vi "create_listener.vi"(0 "control_endpoint":string="tcp://0.0.0.0:5556", 5 "Port":string="5555", 7 "recv_timout_default_ms":dbl=2000.0 format="%#_13g", 9 "send_timout_default_ms":dbl=2000.0 format="%#_13g", 11 "error in (no error)":errorcluster) -> (4 "zmq_mlt out":refnum<class "zmq_multipart_lib.lvclass">, 15 "error out":errorcluster)   [LabVIEW 2019, in "zmq_multipart_lib.lvlib" / "zmq_multipart_lib.lvclass"]
uses:
  zmq_multipart_lib.lvclass
  <vilib>/addons/zeromq/socket_type.ctl
  zmq_multipart_lib.lvclass/zmq_multipart_lib.ctl
  <vilib>/addons/zeromq/zmq_context.lvclass
  <vilib>/addons/zeromq/zmq_socket.lvclass
  <vilib>/addons/zeromq/zeromq.lvlib
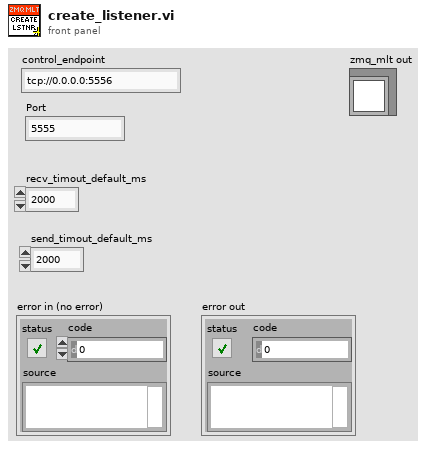
[diagram p1: front panel]
types:
  T1 = typedef "zeromq.lvlib/socket_type.ctl" = enum8{"ZMQ_PAIR", "ZMQ_PUB", "ZMQ_SUB", "ZMQ_REQ", "ZMQ_REP", "ZMQ_DEALER", "ZMQ_ROUTER", "ZMQ_PULL", "ZMQ_PUSH", "ZMQ_XPUB", "ZMQ_XSUB"}
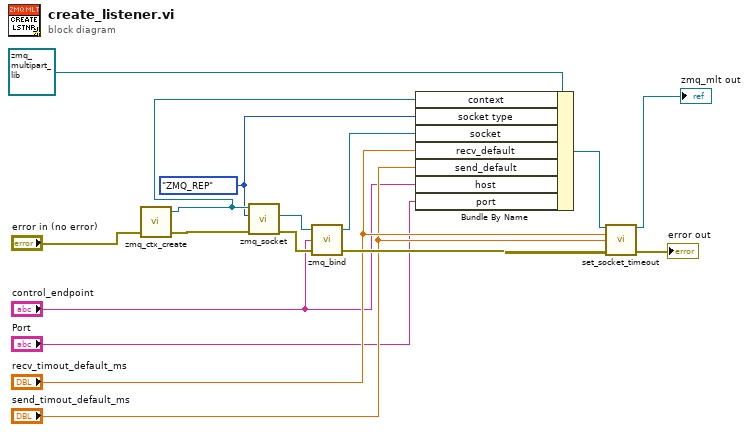
[diagram p0: block diagram]
diagram:
  w7 = socket_type."ZMQ_REP" ("socket type")
  n1 = call <vilib>:"zmq_ctx_create.vi"("error in"="error in (no error)") -> ("error out"=w12:errorcluster, "context out"=w10:refnum<class "zmq_context.lvclass">)  [unwired: 3 in]
  n2 = call <vilib>:"zmq_socket.vi"("error in"=w12, "socket type"=w7, "context in"=w10) -> ("error out"=w14:errorcluster, "socket out"=w6:refnum<class "zmq_socket.lvclass">)  [unwired: 2 in, 1 out]
  n3 = call <vilib>:"zmq_bind.vi"("error in"=w14, "endpoint"="control_endpoint", "socket in"=w6) -> ("error out"=w15:errorcluster, "socket out"=w5:refnum<class "zmq_socket.lvclass">)  [unwired: 1 in]
  n4 = Bundle By Name(cluster=refnum<class "zmq_multipart_lib.lvclass"> refnum ("zmq_mlt in"), "context"=w10, "socket type"=w7, "socket"=w5, "recv_default"="recv_timout_default_ms", "send_default"="send_timout_default_ms", "host"="control_endpoint", "port"="Port") -> (w9:refnum<class "zmq_multipart_lib.lvclass">)
  n5 = call "set_socket_timeout.vi"("zmq_mlt in"=w9, "recv_timeout_ms"="recv_timout_default_ms", "send_timeout_ms"="send_timout_default_ms", "error in (no error)"=w15) -> ("zmq_mlt out"=→"zmq_mlt out":refnum<class "zmq_multipart_lib.lvclass">, "error out"=→"error out":errorcluster)  [unwired: 10 in]
